vi "interpola grafico.vi"(8 "graph ref":refnum<vi>, 9 "Interpola":refnum<vi>, 11 "Array":cluster{"X":dbl[], "Y":dbl[]}[](array[cluster])) -> (3 "Array out":cluster{"X":dbl[], "Y":dbl[]}[](array[cluster]))   [LabVIEW 2019]
uses:
  <vilib>/Analysis/1siggen.llb/Ramp Pattern by Samples.vi
  <vilib>/Analysis/NI_AALPro.lvlib
  <vilib>/Analysis/NI_AALBase.lvlib
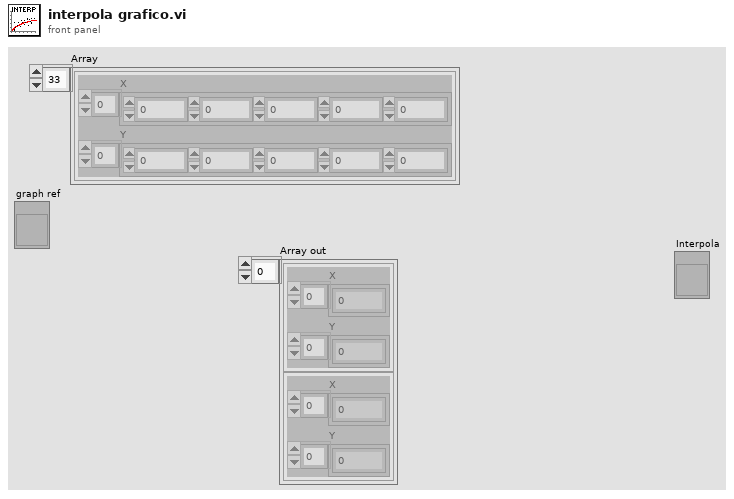
[diagram p1: front panel]
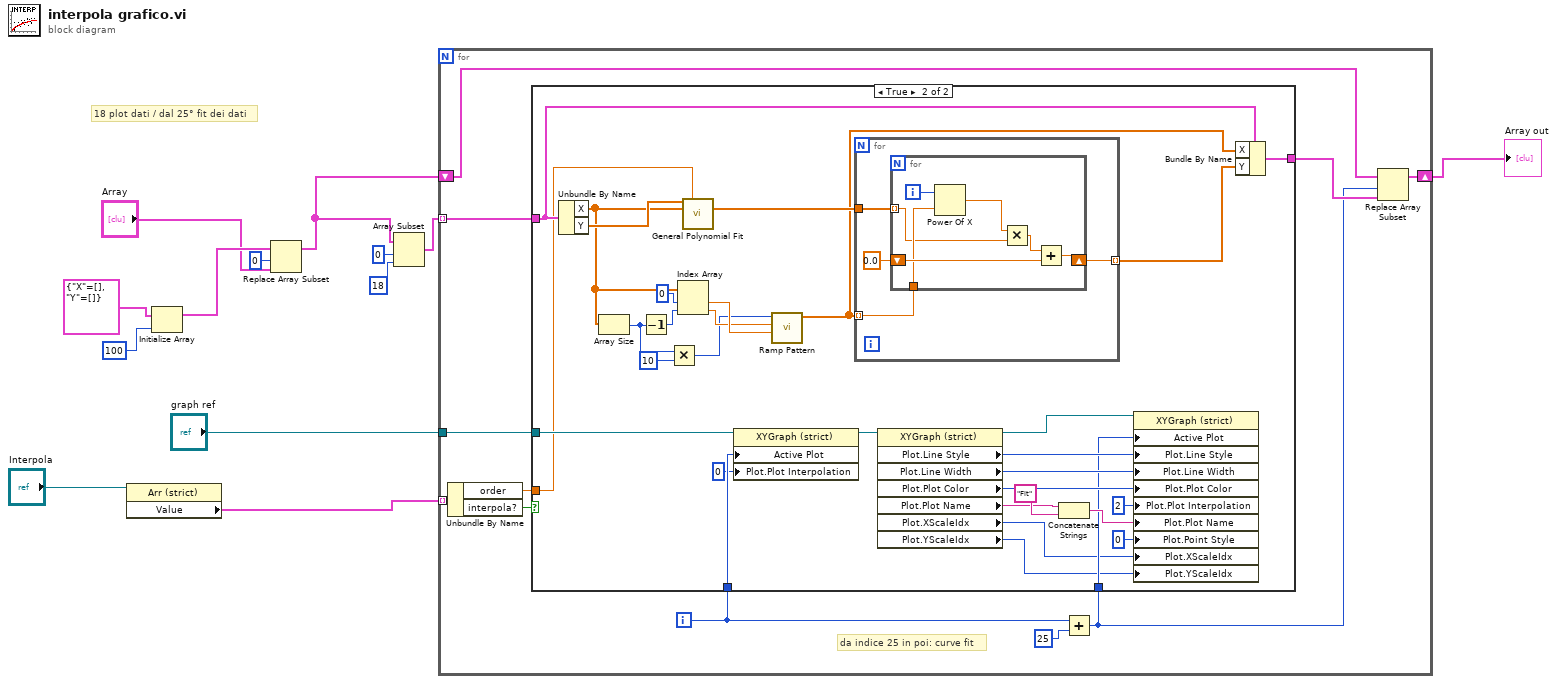
[diagram p0: block diagram]
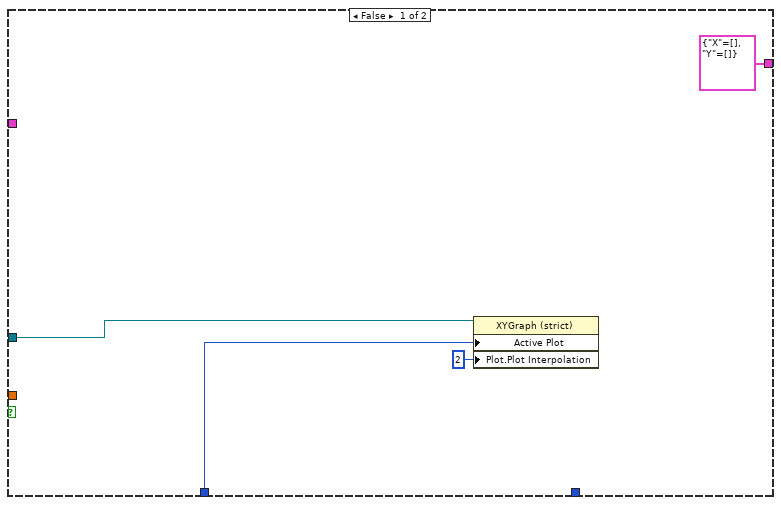
[diagram p2: hidden frame]
diagram:
  # "18 plot dati / dal 25° fit dei dati"
  n1 = property class="Arr (strict)"(reference="Interpola") -> ("Value"=w10:cluster{"interpola?":bool, "order":dbl}[])  [unwired: 1 in, 2 out]
  n2 = Initialize Array(cluster{"X":dbl[], "Y":dbl[]} {"X"=[], "Y"=[]} ("QP"), 100 ("dimension size")) -> (w4:cluster{"X":dbl[], "Y":dbl[]}[])
  n3 = Replace Array Subset(array=w4, new element="Array", index=0) -> (w1:cluster{"X":dbl[], "Y":dbl[]}[])
  n4 = Array Subset(array=w1, index=0, length=18) -> (w8:cluster{"X":dbl[], "Y":dbl[]}[])
  n5 = for {
    tunnel: w8 -> [w24] mode=indexing
    shift-right: [w22] -> w13
    shift-left: w1 -> [w21]
    tunnel: "graph ref" -> [w19]
    tunnel: w10 -> [w16] mode=indexing
    i -> [w17]
    # "da indice 25 in poi: curve fit"
    n6 = Unbundle By Name(w16) -> ("order"=w14:dbl, "interpola?"=w15:bool)
    n7 = Add(x=w17, y=25) -> (x+y=w18:i32)
    n8 = case shown="True" w15 {
      tunnel: w24 -> [_ w52]
      tunnel: [cluster{"X":dbl[], "Y":dbl[]} {"X"=[], "Y"=[]} ("QP") w46] -> w20
      tunnel: w19 -> [w27 w36]
      tunnel: w18 -> [_ w35]
      tunnel: w17 -> [w25 w34]
      tunnel: w14 -> [_ w33]
      frame False {
        n9 = property class="XYGraph (strict)"(reference=w27, "Active Plot"=w25, "Plot.Plot Interpolation"=u8 2) -> ()  [unwired: 1 in, 2 out]
      }
      frame True {
        n10 = Unbundle By Name(w52) -> ("X"=w47:dbl[], "Y"=w48:dbl[])
        n11 = Array Size(array=w47) -> (size(s)=w55:i32)
        n12 = Decrement(x=w55) -> (x-1=w58:i32)
        n13 = Multiply(x=w55, y=10) -> (x*y=w53:i32)
        n14 = Index Array(array=w47, index #1=0 ("index"), index #2=w58) -> (element #1=w57:dbl, element #2=w56:dbl)
        n15 = call <vilib>:"General Polynomial Fit.vi"("Y"=w48, "polynomial order"=w33, "X"=w47) -> ("Polynomial Coefficients"=w51:dbl[])  [unwired: 9 in, 3 out]
        n16 = property class="XYGraph (strict)"(reference=w36, "Active Plot"=w34, "Plot.Plot Interpolation"=u8 0) -> (reference out=w37:refnum<vi>)  [unwired: 1 in, 1 out]
        n17 = call-poly <vilib>:"Ramp Pattern.vi"("start"=w57, "end"=w56, "samples"=w53) -> ("Ramp Pattern"=w50:dbl[])  [unwired: 7 in, 1 out]
        n18 = for {
          tunnel: w51 -> [w63]
          tunnel: [w61] -> w49 mode=indexing
          tunnel: w50 -> [w60] mode=indexing
          n19 = for {
            tunnel: w63 -> [w64] mode=indexing
            tunnel: w60 -> [w65]
            shift-right: [w68] -> w61
            shift-left: 0.0 -> [w67]
            i -> [w66]
            n20 = Power Of X(1:w65, 2:w66) -> (0:w70:dbl)
            n21 = Multiply(x=w70, y=w64) -> (x*y=w69:dbl)
            n22 = Add(x=w69, y=w67) -> (x+y=w68:dbl)
          }
        }
        n23 = property class="XYGraph (strict)"(reference=w37) -> (reference out=w38:refnum<vi>, "Plot.Line Style"=w40:u8, "Plot.Line Width"=w41:u8, "Plot.Plot Color"=w42:u32, "Plot.Plot Name"=w43:string, "Plot.XScaleIdx"=w30:u32, "Plot.YScaleIdx"=w29:u32)  [unwired: 1 in, 1 out]
        n24 = Concatenate Strings(w43, "Fit" ("string")) -> (w45:string)
        n25 = property class="XYGraph (strict)"(reference=w38, "Active Plot"=w35, "Plot.Line Style"=w40, "Plot.Line Width"=w41, "Plot.Plot Color"=w42, "Plot.Plot Interpolation"=u8 2, "Plot.Plot Name"=w45, "Plot.Point Style"=u8 0, "Plot.XScaleIdx"=w30, "Plot.YScaleIdx"=w29) -> ()  [unwired: 1 in, 2 out]
        n26 = Bundle By Name(cluster=w52, "X"=w50, "Y"=w49) -> (w46:cluster{"X":dbl[], "Y":dbl[]})
      }
    }
    n27 = Replace Array Subset(array=w21, new element=w20, index=w18) -> (w22:cluster{"X":dbl[], "Y":dbl[]}[])
  }
  "Array out" <- w13
